vi "Oxford Read Channel -- Hg.vi"(6 "milliseconds -- wait time":u32=11, 8 "error in (no error)":errorcluster, 10 "Channel #":i32=1, 11 "VISA resource name":refnum<visa-resource-name>) -> (0 "error out":errorcluster, 1 "read buffer":string, 2 "Data":dbl, 3 "VISA resource name out":refnum<visa-resource-name>)   [LabVIEW 2015]
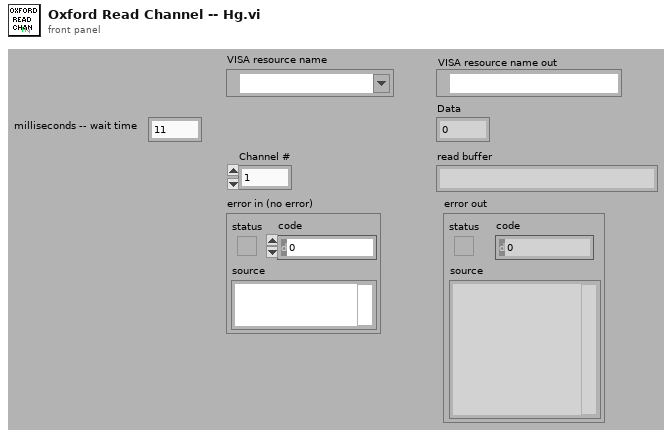
[diagram p1: front panel]
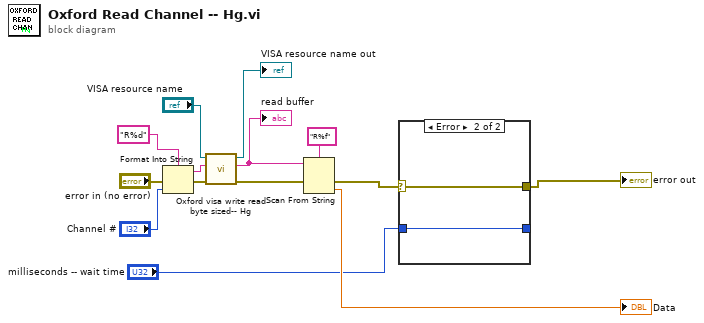
[diagram p0: block diagram]
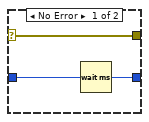
[diagram p2: hidden frame]
diagram:
  n1 = Format Into String(format string="R%d" ("write buffer"), error in="error in (no error)", "Channel #") -> (resulting string=w8:string, error out=w11:errorcluster)  [unwired: 1 in]
  n2 = call "Oxford visa write read byte sized-- Hg.vi"("error in (no error)"=w11, "write buffer"=w8, "VISA resource name"="VISA resource name") -> ("error out"=w7:errorcluster, "read buffer"=w4:string, "VISA resource name out"=→"VISA resource name out":refnum<visa-resource-name>)  [unwired: 6 in]
  "read buffer" <- w4
  n3 = Scan From String(format string="R%f", input string=w4, error in=w7) -> (error out=w3:errorcluster, output 1=→"Data":dbl)  [unwired: 2 in, 2 out]
  n4 = case shown="Error" w3 {
    selector: w3 -> [w17 w19]
    tunnel: [w17 w19] -> w2
    tunnel: [w16 w18] -> _
    tunnel: "milliseconds -- wait time" -> [w15 w18]
    frame No Error {
      n5 = Wait (ms)(milliseconds to wait=w15) -> (millisecond timer value=w16:u32)
    }
    frame Error {
    }
  }
  "error out" <- w2
